vi "StringHeaderToCluster(SubVI).vi"(8 "error in":errorcluster, 10 "UNDT_Cluster in":T1 {"Gain Coeff" format="%#_6e"; "Reserve 1" format="%02x"; "Mux TX" format="%02x"; "Mux RX" format="%02x"; "ScanDelay" format="%02x"; "PacketCounter" format="%08x"; "SamplingInterval" format="%#_6e"; "Lose Packet" format="%08x"; "EncodersParam2" format="%016x"; "EncodersParam1" format="%016x"; "CRC 8" format="%02x"; "N chanel" format="%02x"; "N tick" format="%02x"; "Ncycle" format="%04x"; "FrameFormatVersion" format="%02x"; "MagicWord" format="%.0x"}, 11 "string in":string) -> (0 "error out":errorcluster, 2 "UNDT_Cluster out":T1 {"Gain Coeff" format="%#_6e"; "Reserve 1" format="%02x"; "Mux TX" format="%02x"; "Mux RX" format="%02x"; "ScanDelay" format="%02x"; "PacketCounter" format="%08x"; "SamplingInterval" format="%#_6e"; "Lose Packet" format="%08x"; "EncodersParam2" format="%016x"; "EncodersParam1" format="%016x"; "CRC 8" format="%02x"; "N chanel" format="%02x"; "N tick" format="%02x"; "Ncycle" format="%04x"; "FrameFormatVersion" format="%02x"; "MagicWord" format="%.0x"})   [LabVIEW 2017]
uses:
  Control_EU/UNDT_ClusterPack (Type).ctl
  <vilib>/Utility/error.llb/DialogType.ctl
panel:
  out "*(type *) &x":u32 format="%x"
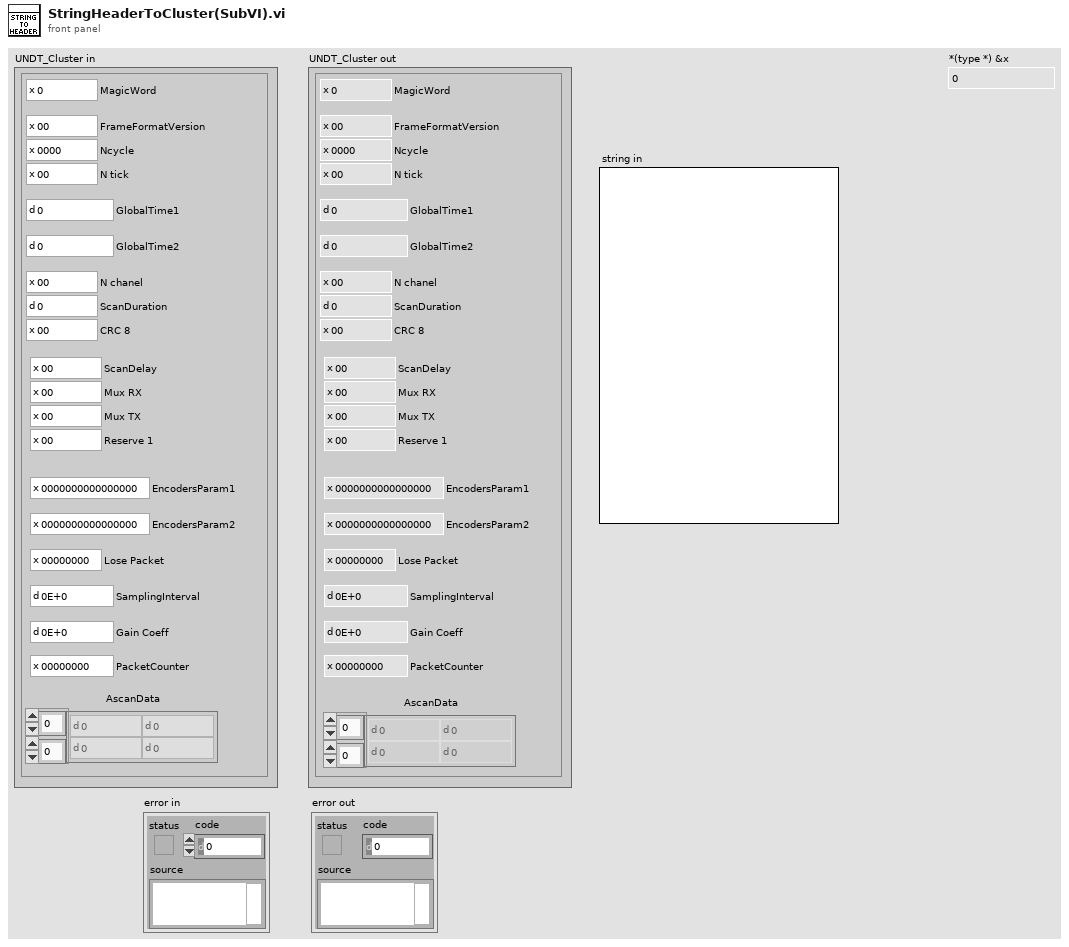
[diagram p1: front panel]
types:
  T1 = typedef "UNDT_ClusterPack (Type).ctl" = cluster{"MagicWord":u32, "FrameFormatVersion":u8, "Ncycle":u16, "N tick":u8, "GlobalTime1":u32, "GlobalTime2":u32, "N chanel":u8, "ScanDuration":u16, "CRC 8":u8, "EncodersParam1":u64, "EncodersParam2":u64, "Lose Packet":u32, "SamplingInterval":sgl, "PacketCounter":u32, "AscanData":dbl[][], "ScanDelay":u16, "Mux RX":u8, "Mux TX":u8, "Reserve 1":u8, "Gain Coeff":sgl}
  T2 = typedef "DialogType.ctl" = u16
  T3 = enum16{"big-endian, network order", "native, host order", "little-endian"}
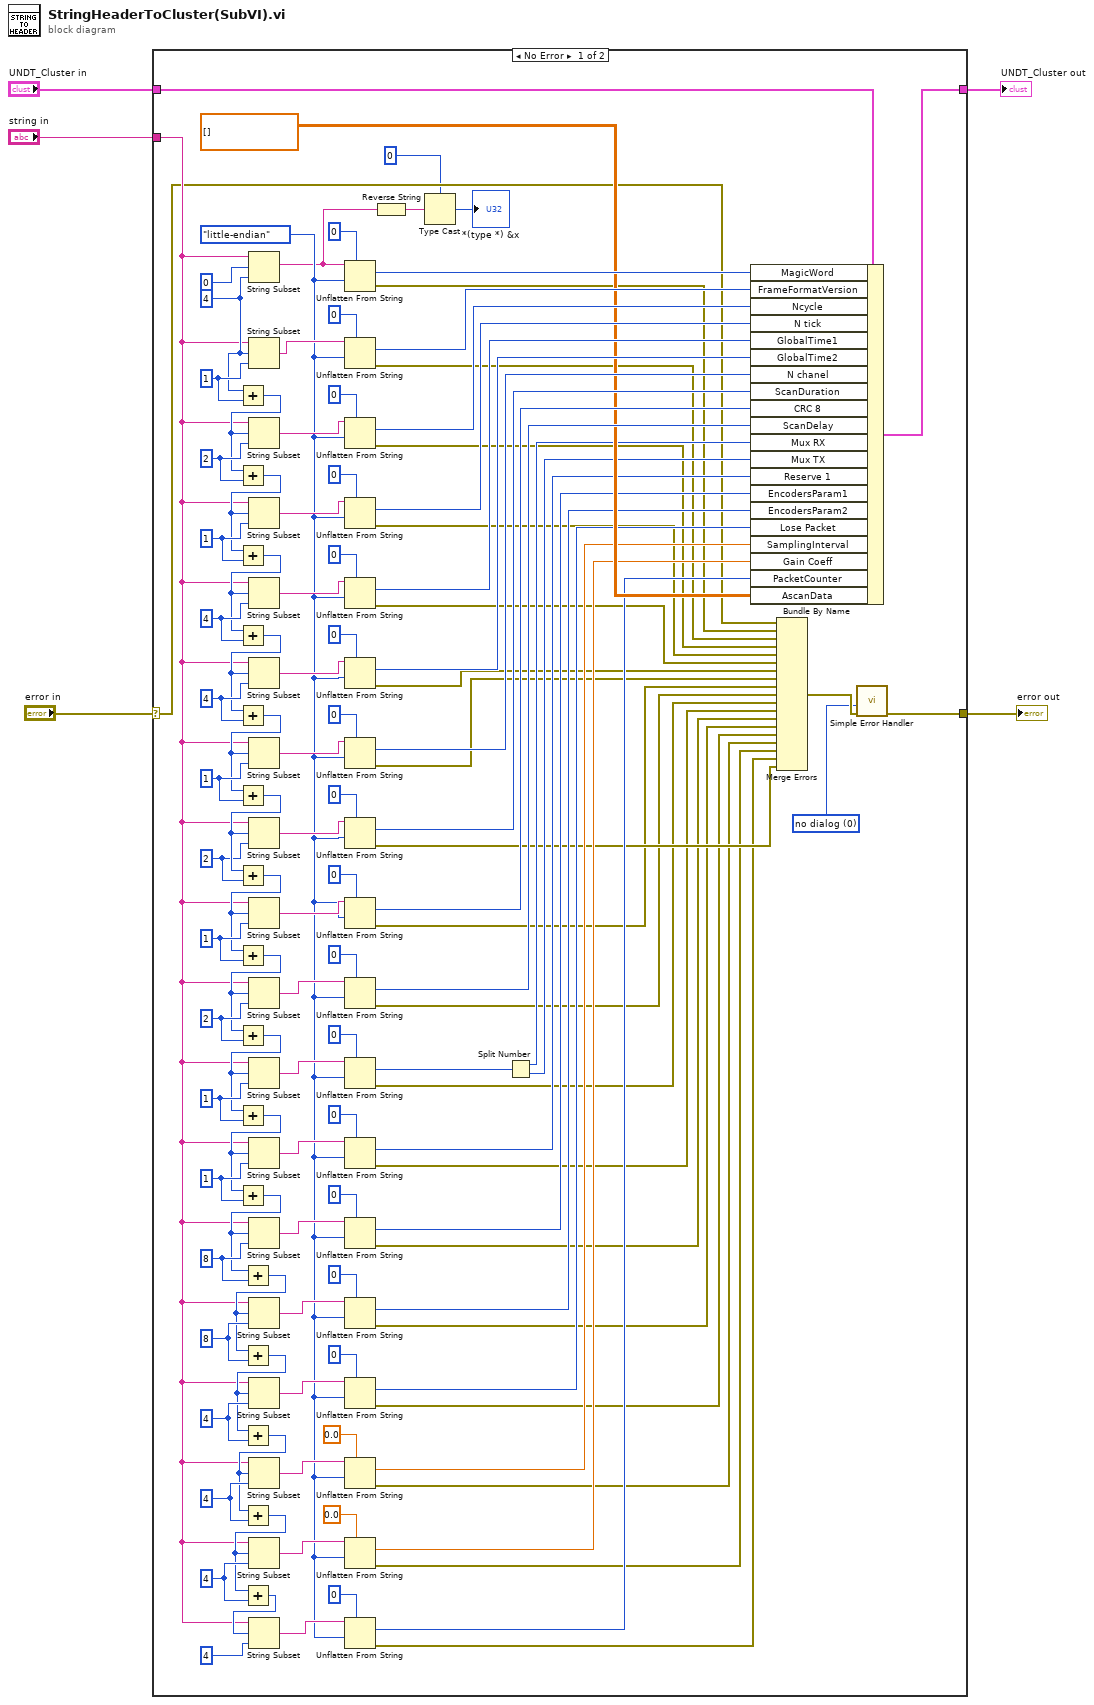
[diagram p0: block diagram]
diagram:
  n1 = case shown="No Error" "error in" {
    selector: "error in" -> [w31 w127]
    tunnel: "UNDT_Cluster in" -> [w57 w128]
    tunnel: [w56 w128] -> w4
    tunnel: "string in" -> [w33 _]
    tunnel: [w10 w127] -> w1
    frame No Error {
      w11 = T2 0 items=["no dialog", "OK message", "continue or stop message", "OK message + warnings", "continue/stop + warnings"] ("type of dialog (OK msg:1)")
      w124 = 4 ("length (rest)")
      w122 = 4 ("length (rest)")
      w118 = 4 ("length (rest)")
      w114 = 8 ("length (rest)")
      w112 = 8 ("length (rest)")
      w107 = 1 ("length (rest)")
      w101 = 1 ("length (rest)")
      w98 = 2 ("length (rest)")
      w91 = 1 ("length (rest)")
      w88 = 2 ("length (rest)")
      w85 = 1 ("length (rest)")
      w81 = 4 ("length (rest)")
      w125 = 4 ("length (rest)")
      w76 = 1 ("length (rest)")
      w68 = 2 ("length (rest)")
      w63 = 1 ("length (rest)")
      w32 = T3."little-endian" ("byte order (0:big-endian, network order)")
      w62 = 4 ("length (rest)")
      n2 = Add(x=w62, y=w63) -> (x+y=w67:i32)
      n3 = Add(x=w67, y=w68) -> (x+y=w71:i32)
      n4 = Add(x=w71, y=w76) -> (x+y=w75:i32)
      n5 = Add(x=w75, y=w125) -> (x+y=w80:i32)
      n6 = Add(x=w80, y=w81) -> (x+y=w84:i32)
      n7 = Add(x=w84, y=w85) -> (x+y=w89:i32)
      n8 = Add(x=w89, y=w88) -> (x+y=w90:i32)
      n9 = Add(x=w90, y=w91) -> (x+y=w97:i32)
      n10 = Add(x=w97, y=w98) -> (x+y=w100:i32)
      n11 = Add(x=w100, y=w101) -> (x+y=w103:i32)
      n12 = Add(x=w103, y=w107) -> (x+y=w106:i32)
      n13 = Add(x=w106, y=w112) -> (x+y=w113:i32)
      n14 = Add(x=w113, y=w114) -> (x+y=w117:i32)
      n15 = Add(x=w117, y=w118) -> (x+y=w121:i32)
      n16 = Add(x=w121, y=w122) -> (x+y=w123:i32)
      n17 = Add(x=w123, y=w124) -> (x+y=w38:i32)
      n18 = String Subset(string=w33, offset (0)=0, length (rest)=w62) -> (substring=w7:string)
      n19 = String Subset(string=w33, offset (0)=w62, length (rest)=w63) -> (substring=w61:string)
      n20 = String Subset(string=w33, offset (0)=w67, length (rest)=w68) -> (substring=w65:string)
      n21 = String Subset(string=w33, offset (0)=w71, length (rest)=w76) -> (substring=w66:string)
      n22 = String Subset(string=w33, offset (0)=w75, length (rest)=w125) -> (substring=w70:string)
      n23 = String Subset(string=w33, offset (0)=w80, length (rest)=w81) -> (substring=w74:string)
      n24 = String Subset(string=w33, offset (0)=w84, length (rest)=w85) -> (substring=w77:string)
      n25 = String Subset(string=w33, offset (0)=w89, length (rest)=w88) -> (substring=w83:string)
      n26 = String Subset(string=w33, offset (0)=w90, length (rest)=w91) -> (substring=w86:string)
      n27 = String Subset(string=w33, offset (0)=w97, length (rest)=w98) -> (substring=w93:string)
      n28 = String Subset(string=w33, offset (0)=w100, length (rest)=w101) -> (substring=w95:string)
      n29 = String Subset(string=w33, offset (0)=w103, length (rest)=w107) -> (substring=w104:string)
      n30 = String Subset(string=w33, offset (0)=w106, length (rest)=w112) -> (substring=w105:string)
      n31 = String Subset(string=w33, offset (0)=w113, length (rest)=w114) -> (substring=w109:string)
      n32 = String Subset(string=w33, offset (0)=w117, length (rest)=w118) -> (substring=w110:string)
      n33 = String Subset(string=w33, offset (0)=w121, length (rest)=w122) -> (substring=w116:string)
      n34 = String Subset(string=w33, offset (0)=w123, length (rest)=w124) -> (substring=w119:string)
      n35 = String Subset(string=w33, offset (0)=w38, length (rest)=4 ("length (rest)")) -> (substring=w35:string)
      n36 = Unflatten From String(type=u32 0 ("MagicWord 2"), binary string=w7, byte order (0:big-endian, network order)=w32) -> (value=w55:u32, error out=w30:errorcluster)  [unwired: 2 in, 1 out]
      n37 = Unflatten From String(type=u8 0 ("MagicWord 2"), binary string=w61, byte order (0:big-endian, network order)=w32) -> (value=w54:u8, error out=w29:errorcluster)  [unwired: 2 in, 1 out]
      n38 = Unflatten From String(type=u16 0 ("MagicWord 2"), binary string=w65, byte order (0:big-endian, network order)=w32) -> (value=w53:u16, error out=w28:errorcluster)  [unwired: 2 in, 1 out]
      n39 = Unflatten From String(type=u8 0 ("MagicWord 2"), binary string=w66, byte order (0:big-endian, network order)=w32) -> (value=w52:u8, error out=w27:errorcluster)  [unwired: 2 in, 1 out]
      n40 = Unflatten From String(type=u32 0 ("MagicWord 2"), binary string=w70, byte order (0:big-endian, network order)=w32) -> (value=w51:u32, error out=w26:errorcluster)  [unwired: 2 in, 1 out]
      n41 = Unflatten From String(type=u32 0 ("MagicWord 2"), binary string=w74, byte order (0:big-endian, network order)=w32) -> (value=w50:u32, error out=w25:errorcluster)  [unwired: 2 in, 1 out]
      n42 = Unflatten From String(type=u8 0 ("MagicWord 2"), binary string=w77, byte order (0:big-endian, network order)=w32) -> (value=w79:u8, error out=w24:errorcluster)  [unwired: 2 in, 1 out]
      n43 = Unflatten From String(type=u16 0 ("MagicWord 2"), binary string=w83, byte order (0:big-endian, network order)=w32) -> (value=w126:u16, error out=w23:errorcluster)  [unwired: 2 in, 1 out]
      n44 = Unflatten From String(type=u8 0 ("MagicWord 2"), binary string=w86, byte order (0:big-endian, network order)=w32) -> (value=w49:u8, error out=w22:errorcluster)  [unwired: 2 in, 1 out]
      n45 = Unflatten From String(type=u16 0 ("MagicWord 2"), binary string=w93, byte order (0:big-endian, network order)=w32) -> (value=w94:u16, error out=w21:errorcluster)  [unwired: 2 in, 1 out]
      n46 = Unflatten From String(type=u8 0 ("MagicWord 2"), binary string=w95, byte order (0:big-endian, network order)=w32) -> (value=w47:u8, error out=w20:errorcluster)  [unwired: 2 in, 1 out]
      n47 = Unflatten From String(type=u8 0 ("MagicWord 2"), binary string=w104, byte order (0:big-endian, network order)=w32) -> (value=w44:u8, error out=w19:errorcluster)  [unwired: 2 in, 1 out]
      n48 = Unflatten From String(type=u64 0 ("MagicWord 2"), binary string=w105, byte order (0:big-endian, network order)=w32) -> (value=w43:u64, error out=w18:errorcluster)  [unwired: 2 in, 1 out]
      n49 = Unflatten From String(type=u64 0 ("MagicWord 2"), binary string=w109, byte order (0:big-endian, network order)=w32) -> (value=w42:u64, error out=w17:errorcluster)  [unwired: 2 in, 1 out]
      n50 = Unflatten From String(type=u32 0 ("MagicWord 2"), binary string=w110, byte order (0:big-endian, network order)=w32) -> (value=w41:u32, error out=w16:errorcluster)  [unwired: 2 in, 1 out]
      n51 = Unflatten From String(type=sgl 0.0 ("MagicWord 2"), binary string=w116, byte order (0:big-endian, network order)=w32) -> (value=w40:sgl, error out=w15:errorcluster)  [unwired: 2 in, 1 out]
      n52 = Unflatten From String(type=sgl 0.0 ("MagicWord 2"), binary string=w119, byte order (0:big-endian, network order)=w32) -> (value=w39:sgl, error out=w14:errorcluster)  [unwired: 2 in, 1 out]
      n53 = Unflatten From String(type=u32 0 ("MagicWord 2"), binary string=w35, byte order (0:big-endian, network order)=w32) -> (value=w34:u32, error out=w13:errorcluster)  [unwired: 2 in, 1 out]
      n54 = Reverse String(1:w7) -> (0:w6:string)
      n55 = Type Cast(type=u32 0 ("MagicWord 2"), x=w6) -> (*(type *) &x=→"*(type *) &x":u32)
      n56 = Split Number(x=w47) -> (hi(x)=w46:u8, lo(x)=w45:u8)
      n57 = Bundle By Name(cluster=w57, "MagicWord"=w55, "FrameFormatVersion"=w54, "Ncycle"=w53, "N tick"=w52, "GlobalTime1"=w51, "GlobalTime2"=w50, "N chanel"=w79, "ScanDuration"=w126, "CRC 8"=w49, "ScanDelay"=w94, "Mux RX"=w46, "Mux TX"=w45, "Reserve 1"=w44, "EncodersParam1"=w43, "EncodersParam2"=w42, "Lose Packet"=w41, "SamplingInterval"=w40, "Gain Coeff"=w39, "PacketCounter"=w34, "AscanData"=dbl[][] [] ("Data1")) -> (w56:T1)
      n58 = Merge Errors(w31, w30, w29, w28, w27, w26, w25, w24, w22, w21, w20, w19, w18, w17, w16, w15, w14, w13, w23) -> (w12:errorcluster)
      n59 = call <vilib>:"Simple Error Handler.vi"("type of dialog (OK msg:1)"=w11, "error in (no error)"=w12) -> ("error out"=w10:errorcluster)  [unwired: 3 in, 4 out]
    }
    frame Error {
    }
  }
  "UNDT_Cluster out" <- w4
  "error out" <- w1
